vi "File_checker_and_finder.vi"(2 "Promp if not found":string, 3 "Filename In":path) -> (0 "cancelled":bool, 1 "Filename Out":path)   [LabVIEW 2010]
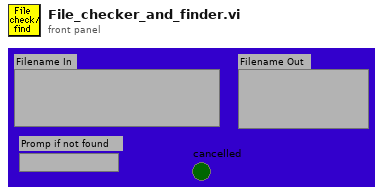
[diagram p1: front panel]
types:
  T1 = enum32{"existing file", "new file", "new or existing file", "existing dir", "new dir", "new or existing dir", "existing file (use LLBs)", "new file (use LLBs)", "new or existing file (use LLBs)", "new or existing file or directory (use LLBs)"}
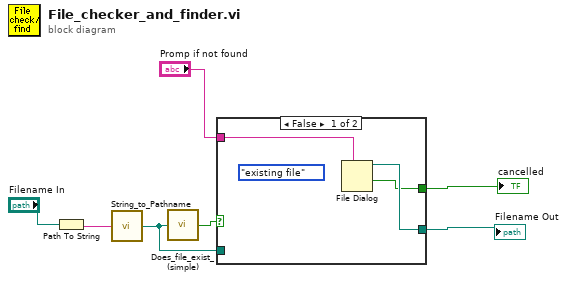
[diagram p0: block diagram]
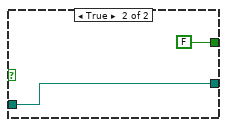
[diagram p2: hidden frame]
diagram:
  n1 = Path To String(path="Filename In") -> (string=w2:string)
  n2 = call "String_to_Pathname.vi"("Input String"=w2) -> ("path"=w1:path)
  n3 = call "Does_file_exist_(simple).vi"("Pathname"=w1) -> ("exists?"=w4:bool)
  n4 = case shown="False" w4 {
    tunnel: "Promp if not found" -> [w10 _]
    tunnel: [w9 w12] -> w7
    tunnel: [w8 FALSE ("cancelled")] -> w5
    tunnel: w1 -> [_ w12]
    frame False {
      (unwired) T1."existing file" ("select mode (2)")
      n5 = File Dialog(7:w10) -> (1:w8:bool, 3:w9:path)  [unwired: 1 in, 7 out]
    }
    frame True {
    }
  }
  "Filename Out" <- w7
  "cancelled" <- w5
